vi "Leggi file opendrive.vi"(11 "file path (dialog if empty)":path=path "C:/Users/TECNICO3-INTESYS/Desktop/opendrive_01_Brs_22p1.pct") -> (0 "Array descriz alarms":string[](array[string]), 1 "Array Name alarms":string[](array[string]), 2 "Array 3":string[][](array[string]))   [LabVIEW 2019]
uses:
  <vilib>/Utility/file.llb/Read From Spreadsheet File (string).vi
panel:
  in  "Array 2":string[](array[string])=["ipa=\"", "um=\"", "scale=\"", "min=\"", "max=\"", "name=\"", "readonly=\"", "typepar=\""]
  in  "Array":string[](array[string])=["ipa=\"", "um=\"", "scale=\"", "min=\"", "max=\"", "descr=\"", "readonly=\"", "typepar=\""]
  # "or"
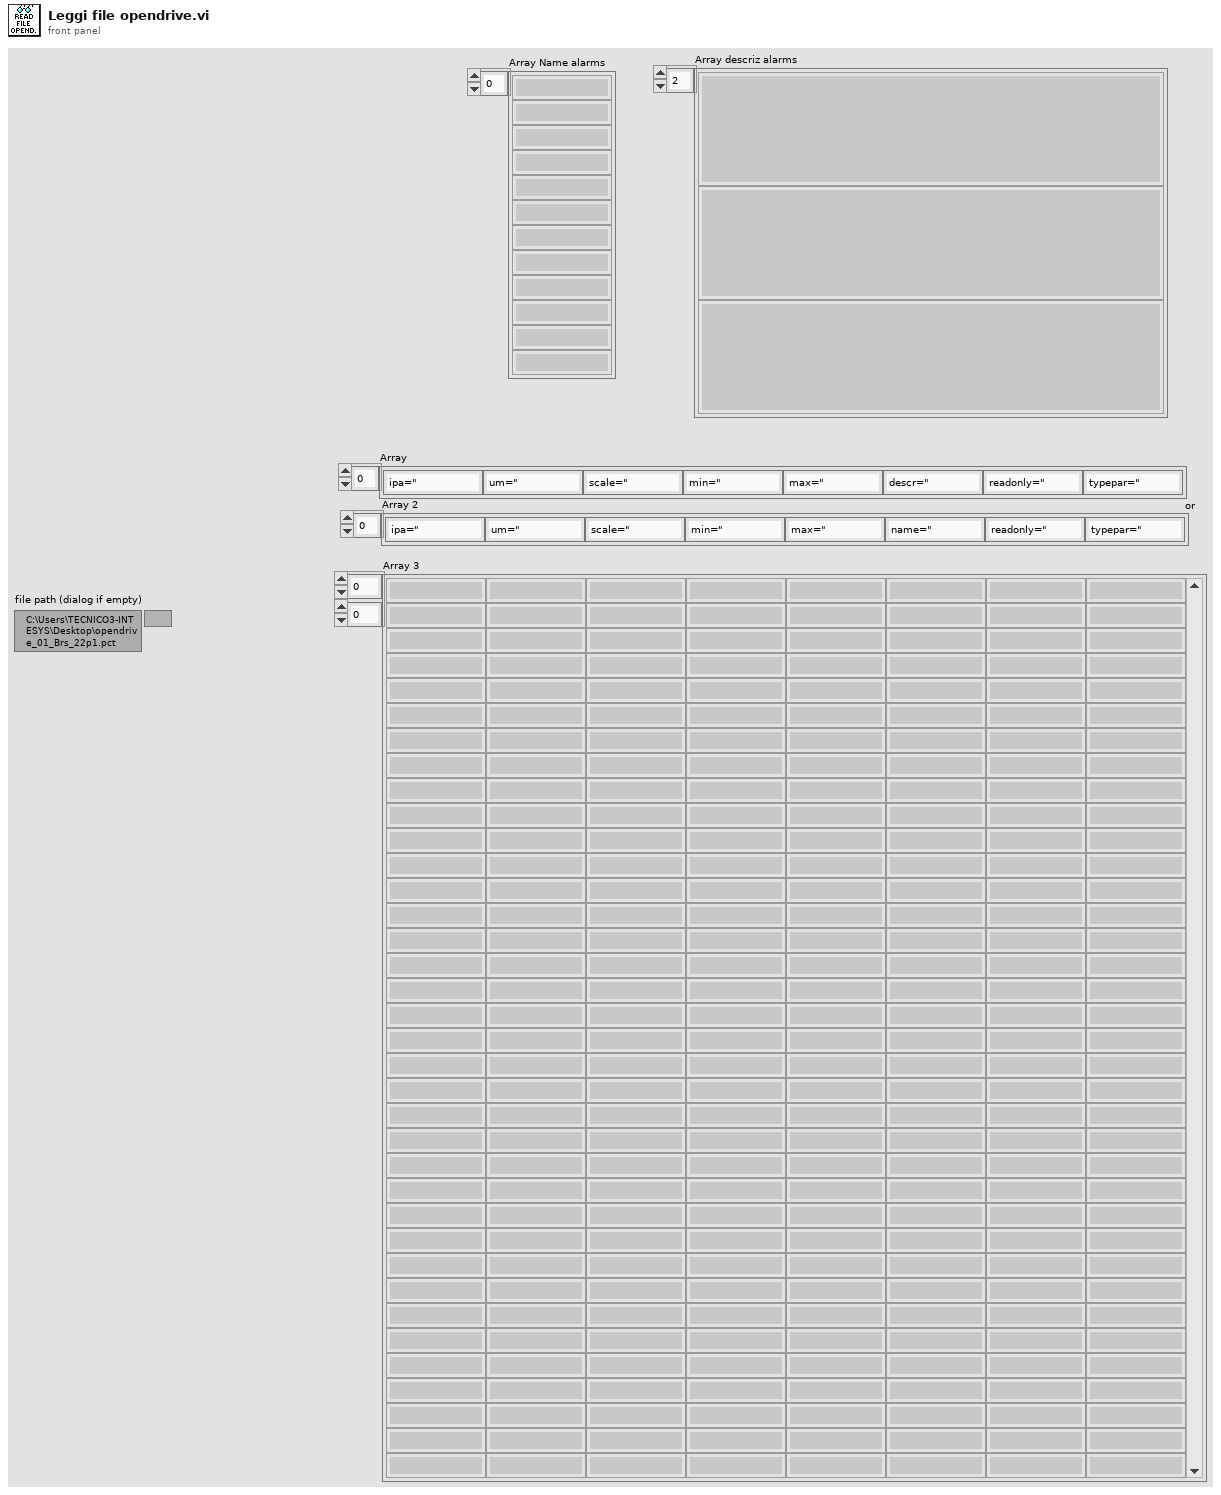
[diagram p1: front panel]
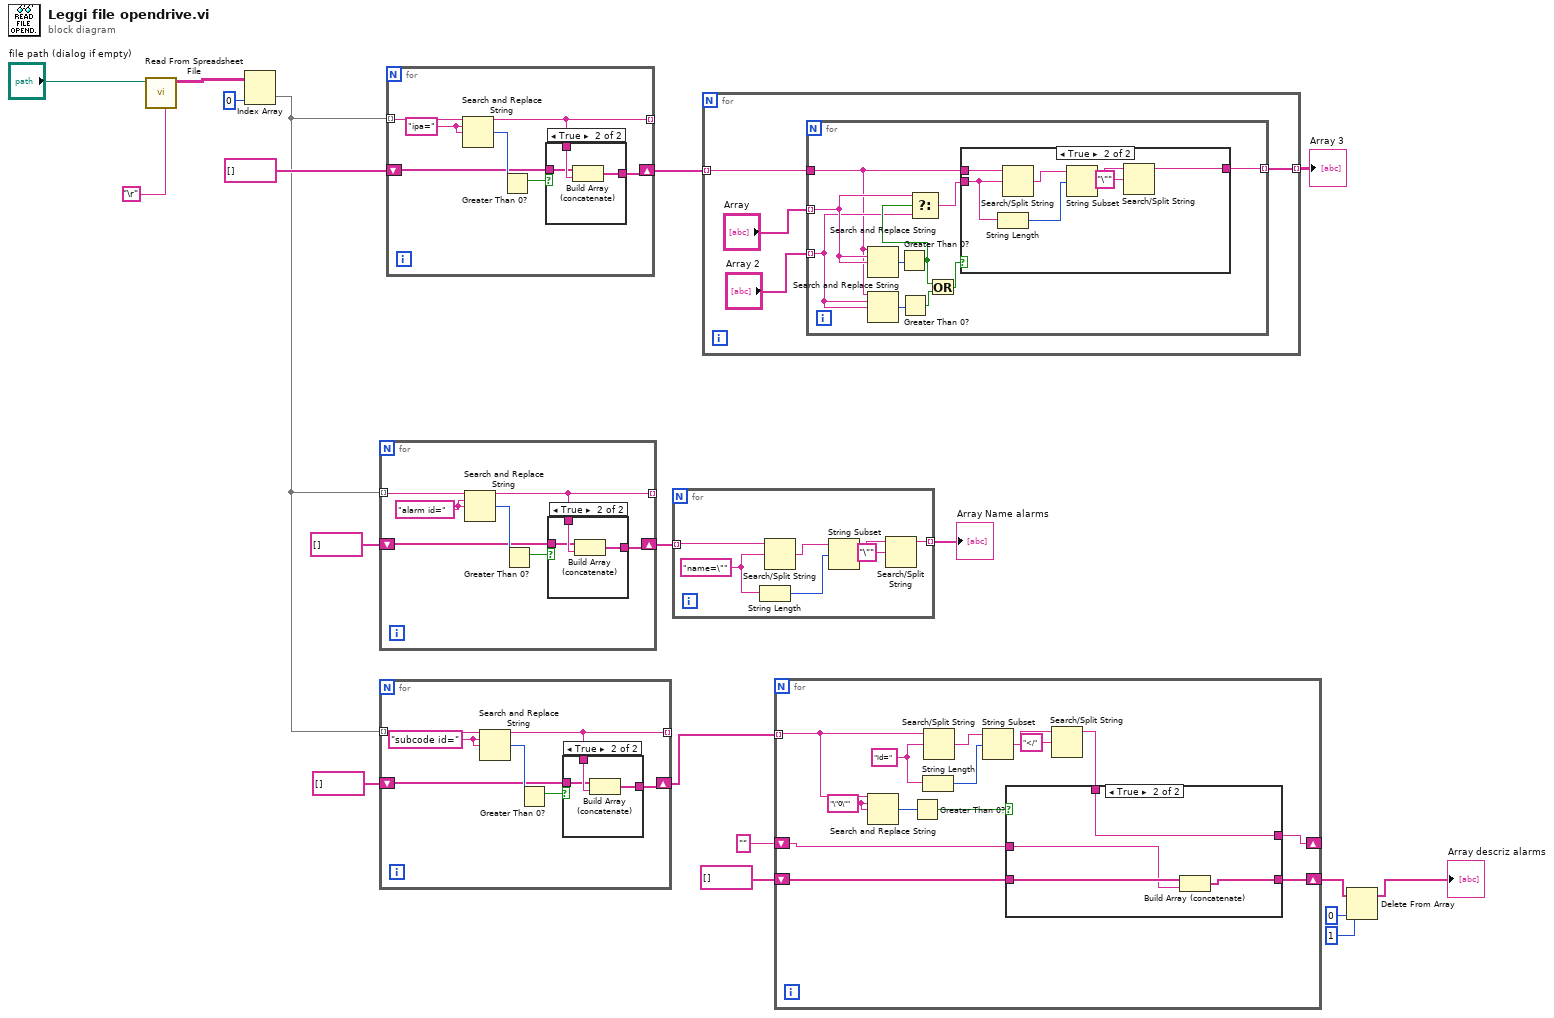
[diagram p0: block diagram]
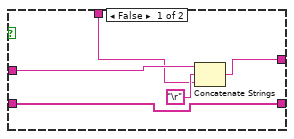
[diagram p2: hidden frame]
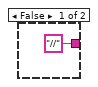
[diagram p5: hidden frame]
diagram:
  n1 = call-poly <vilib>:"Read From Spreadsheet File.vi"("delimiter (\\t)"="\r", "file path (dialog if empty)"="file path (dialog if empty)") -> ("all rows"=w17:string[][])  [unwired: 5 in, 4 out]
  n2 = Index Array(array=w17, index (col)=0 ("disabled index (col)")) -> (element=w10:string[])  [unwired: 1 in]
  n3 = for {
    tunnel: w10 -> [w26] mode=indexing
    tunnel: [w23] -> _ mode=indexing
    shift-right: [w22] -> w9
    shift-left: string[] [] -> [w21]
    w24 = "alarm id=" ("search string")
    n4 = Search and Replace String(input string=w26, search string=w24, replace string=w24) -> (result string=w23:string, number of replacements=w25:i32)  [unwired: 5 in, 2 out]
    n5 = Greater Than 0?(x=w25) -> (x > 0?=w20:bool)
    n6 = case shown="True" w20 {
      tunnel: w23 -> [_ w30]
      tunnel: [w27 w29] -> w22
      tunnel: w21 -> [w27 w28]
      frame False {
      }
      frame True {
        n7 = Build Array (concatenate)(w28, w30) -> (w29:string[])
      }
    }
  }
  n8 = for {
    tunnel: w10 -> [w37] mode=indexing
    tunnel: [w34] -> _ mode=indexing
    shift-right: [w33] -> w7
    shift-left: string[] [] -> [w32]
    w35 = "subcode id=" ("search string")
    n9 = Search and Replace String(input string=w37, search string=w35, replace string=w35) -> (result string=w34:string, number of replacements=w36:i32)  [unwired: 5 in, 2 out]
    n10 = Greater Than 0?(x=w36) -> (x > 0?=w31:bool)
    n11 = case shown="True" w31 {
      tunnel: w34 -> [_ w41]
      tunnel: [w38 w40] -> w33
      tunnel: w32 -> [w38 w39]
      frame False {
      }
      frame True {
        n12 = Build Array (concatenate)(w39, w41) -> (w40:string[])
      }
    }
  }
  n13 = for {
    tunnel: w10 -> [w48] mode=indexing
    tunnel: [w45] -> _ mode=indexing
    shift-right: [w44] -> w14
    shift-left: string[] [] -> [w43]
    w46 = "ipa=" ("search string")
    n14 = Search and Replace String(input string=w48, search string=w46, replace string=w46) -> (result string=w45:string, number of replacements=w47:i32)  [unwired: 5 in, 2 out]
    n15 = Greater Than 0?(x=w47) -> (x > 0?=w42:bool)
    n16 = case shown="True" w42 {
      tunnel: w45 -> [_ w52]
      tunnel: [w49 w51] -> w44
      tunnel: w43 -> [w49 w50]
      frame False {
      }
      frame True {
        n17 = Build Array (concatenate)(w50, w52) -> (w51:string[])
      }
    }
  }
  n18 = for {
    tunnel: w9 -> [w55] mode=indexing
    tunnel: [w53] -> w8 mode=indexing
    w54 = "name=\"" ("string")
    n19 = String Length(string=w54) -> (length=w59:i32)
    n20 = Search/Split String(string=w55, search string/char (-)=w54) -> (match + rest of string=w58:string)  [unwired: 1 in, 2 out]
    n21 = String Subset(string=w58, offset (0)=w59) -> (substring=w57:string)  [unwired: 1 in]
    n22 = Search/Split String(string=w57, search string/char (-)="\"") -> (substring before match=w53:string)  [unwired: 1 in, 2 out]
  }
  "Array Name alarms" <- w8
  n23 = for {
    tunnel: w14 -> [w60] mode=indexing
    tunnel: [w62] -> w13 mode=indexing
    n24 = for {
      tunnel: [w73] -> w62 mode=indexing
      tunnel: "Array" -> [w67] mode=indexing
      tunnel: "Array 2" -> [w65] mode=indexing
      tunnel: w60 -> [w64]
      n25 = Search and Replace String(input string=w64, search string=w67, replace string=w67) -> (number of replacements=w72:i32)  [unwired: 5 in, 3 out]
      n26 = Search and Replace String(input string=w64, search string=w65, replace string=w65) -> (number of replacements=w71:i32)  [unwired: 5 in, 3 out]
      n27 = Greater Than 0?(x=w72) -> (x > 0?=w68:bool)
      n28 = Greater Than 0?(x=w71) -> (x > 0?=w70:bool)
      n29 = Select(t=w67, s=w68, f=w65) -> (s? t:f=w66:string)
      n30 = Or(x=w68, y=w70) -> (x .or. y?=w69:bool)
      n31 = case shown="True" w69 {
        tunnel: ["//" w79] -> w73
        tunnel: w66 -> [_ w76]
        tunnel: w64 -> [_ w75]
        frame False {
        }
        frame True {
          n32 = String Length(string=w76) -> (length=w77:i32)
          n33 = Search/Split String(string=w75, search string/char (-)=w76) -> (match + rest of string=w78:string)  [unwired: 1 in, 2 out]
          n34 = String Subset(string=w78, offset (0)=w77) -> (substring=w80:string)  [unwired: 1 in]
          n35 = Search/Split String(string=w80, search string/char (-)="\"") -> (substring before match=w79:string)  [unwired: 1 in, 2 out]
        }
      }
    }
  }
  "Array 3" <- w13
  n36 = for {
    tunnel: w7 -> [w85] mode=indexing
    shift-right: [w83] -> w4
    shift-left: string[] [] -> [w87]
    shift-right: [w86] -> _
    shift-left: "" -> [w84]
    w90 = "\"0\"" ("search string")
    w91 = "id=" ("string")
    n37 = Search and Replace String(input string=w85, search string=w90, replace string=w90) -> (number of replacements=w89:i32)  [unwired: 5 in, 3 out]
    n38 = Greater Than 0?(x=w89) -> (x > 0?=w88:bool)
    n39 = String Length(string=w91) -> (length=w95:i32)
    n40 = Search/Split String(string=w85, search string/char (-)=w91) -> (match + rest of string=w94:string)  [unwired: 1 in, 2 out]
    n41 = String Subset(string=w94, offset (0)=w95) -> (substring=w93:string)  [unwired: 1 in]
    n42 = Search/Split String(string=w93, search string/char (-)="</") -> (substring before match=w82:string)  [unwired: 1 in, 2 out]
    n43 = case shown="True" w88 {
      tunnel: w87 -> [w97 w104]
      tunnel: [w98 w101] -> w86
      tunnel: w84 -> [w100 w103]
      tunnel: [w97 w102] -> w83
      tunnel: w82 -> [w96 w101]
      frame False {
        n44 = Concatenate Strings(w100, "\r", w96) -> (w98:string)
      }
      frame True {
        n45 = Build Array (concatenate)(w104, w103) -> (w102:string[])
      }
    }
  }
  n46 = Delete From Array(array=w4, length=1, index=0) -> (array with subset deleted=→"Array descriz alarms":string[])  [unwired: 1 out]
